vi "Host_Main.vi"() -> ()   [LabVIEW 2016]
uses:
  <extravilib>/ChannelInstances/Tag-bool/Write With Abort.vi
  <extravilib>/ChannelInstances/High Speed Stream-a[.](u8)/Instantiate.vi
  <extravilib>/ChannelInstances/Tag-bool/Instantiate.vi
  <extravilib>/ChannelInstances/Stream-wfm(dbl)/Instantiate.vi
  <extravilib>/ChannelInstances/Tag-bool/Endpoint.vi
  <vilib>/rtlsdr/rtlsdr.lvlib
  <extravilib>/ChannelInstances/Tag-bool.lvlib
panel:
  in  "stop":bool
  in  "Tuned Frequency (MHz)":u32=101000000 min=87000000 max=105000000 step=100000 format="%.1p"
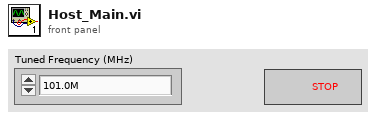
[diagram p1: front panel]
types:
  T1 = typedef "Tag-bool.lvlib/))Channel.ctl" = refnum<queue>
  T2 = typedef "High Speed Stream-a[.](u8).lvlib/)Channel.ctl" = refnum<queue>
  T3 = typedef "Stream-wfm(dbl).lvlib/)Channel.ctl" = refnum<queue>
  T4 = enum32{"invalid app kind", "Development System", "Run Time System", "Student Edition", "Embedded LabVIEW", "Evaluation", "Custom"}
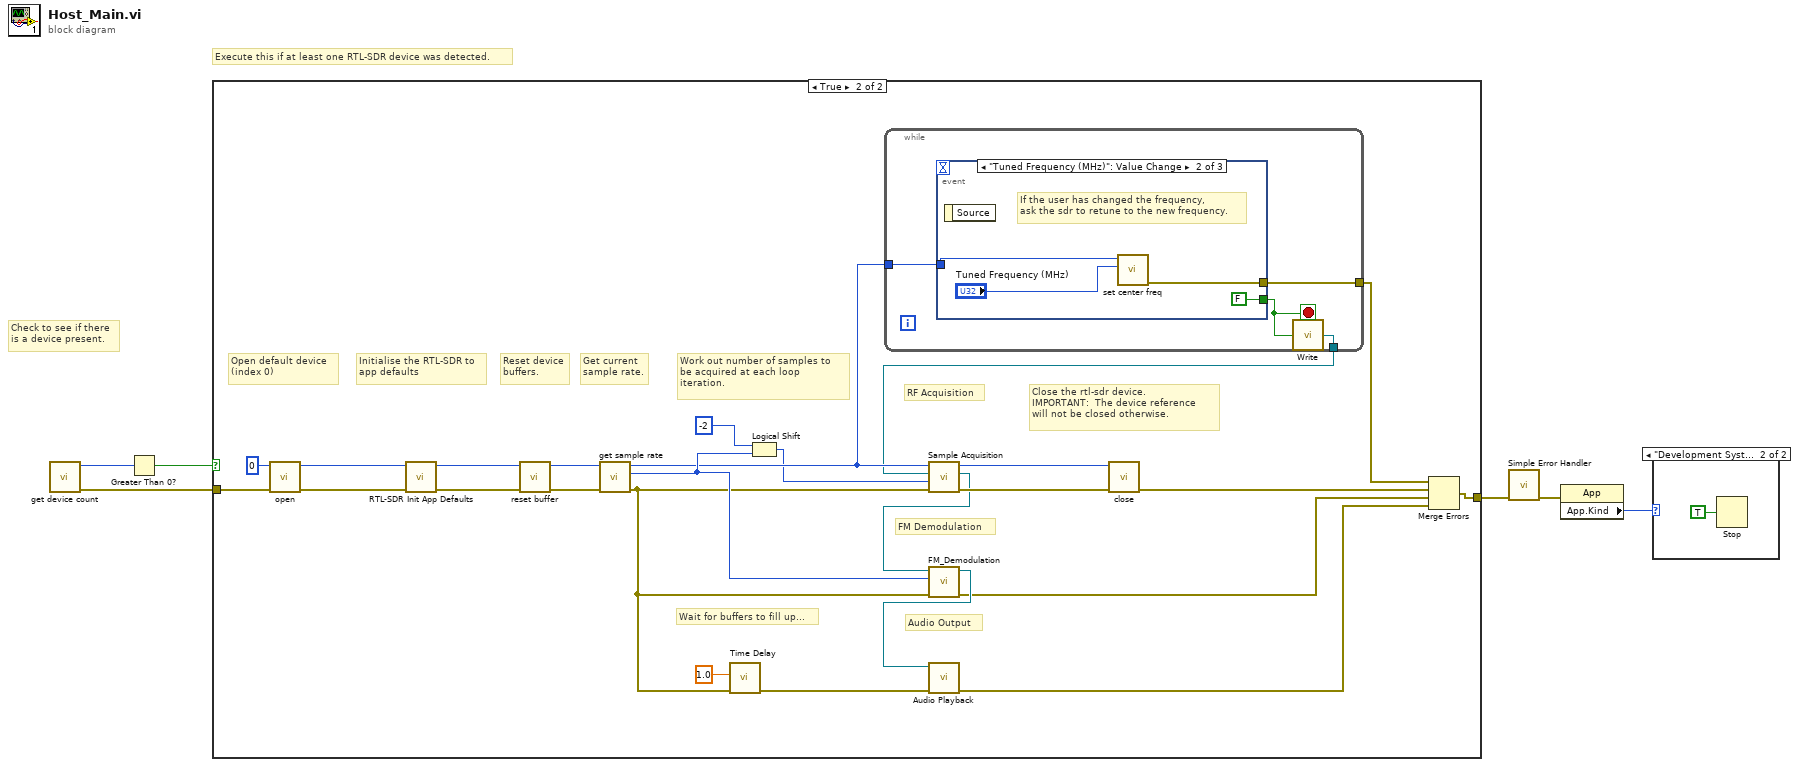
[diagram p0: block diagram]
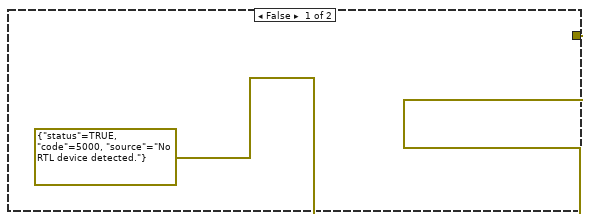
[diagram p2: hidden frame]
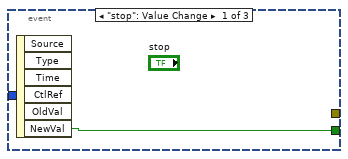
[diagram p3: hidden frame]
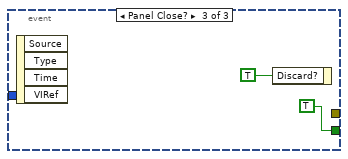
[diagram p4: hidden frame]
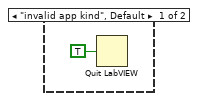
[diagram p5: hidden frame]
diagram:
  # "Execute this if at least one RTL-SDR device was detected."
  # "Check to see if there\nis a device present."
  n1 = call <vilib>:"get device count.vi"() -> ("error out"=w5:errorcluster, "Device Count"=w4:u32)  [unwired: 10 in]
  n2 = Greater Than 0?(x=w4) -> (x > 0?=w3:bool)
  n3 = case shown="True" w3 {
    tunnel: [errorcluster {"status"=TRUE, "code"=5000, "source"="No RTL device detected."} ("error out") w19] -> w6
    tunnel: w5 -> [_ w30]
    frame False {
    }
    frame True {
      # "Wait for buffers to fill up..."
      # "RF Acquisition"
      # "Audio Output"
      # "FM Demodulation"
      # "Reset device\nbuffers."
      # "Get current\nsample rate."
      # "Initialise the RTL-SDR to\napp defaults"
      # "Work out number of samples to\nbe acquired at each loop\niteration."
      # "Close the rtl-sdr device.\nIMPORTANT:  The device reference\nwill not be closed otherwise."
      # "Open default device\n(index 0)"
      n4 = call <vilib>:"open.vi"("error in (no error)"=w30, "Device Index"=u32 0 ("index")) -> ("error out"=w28:errorcluster, "DeviceRefnum Out"=w27:u64)  [unwired: 6 in]
      n5 = call "RTL-SDR Init App Defaults.vi"("error in (no error)"=w28, "RTL-SDR Device In"=w27) -> ("error out"=w26:errorcluster, "RTL-SDR Device Out"=w25:u64)  [unwired: 8 in]
      n6 = call <vilib>:"reset buffer.vi"("error in (no error)"=w26, "DeviceRefnum"=w25) -> ("error out"=w24:errorcluster, "DeviceRefnum Out"=w23:u64)  [unwired: 7 in, 1 out]
      n7 = call <vilib>:"get sample rate.vi"("error in (no error)"=w24, "DeviceRefnum"=w23) -> ("error out"=w10:errorcluster, "Sample Rate (Hz)"=w18:u32, "DeviceRefnum Out"=w16:u64)  [unwired: 7 in]
      n8 = call "Time Delay"("error in (no error)"=w10, "Delay Time (s)"=1.0) -> ("error out"=w9:errorcluster)  [unwired: 9 in]
      n9 = Logical Shift(y=i8 -2, x=w18) -> (x << y=w14:u32)
      n10 = while {
        tunnel: w16 -> [w36]
        tunnel: [w34] -> w15
        tunnel: [w33] -> w11
        stop <- w35 stop-if-true
        n11 = event shown="[1] \"Tuned Frequency (MHz)\": Value Change" {
          selector: _ -> [_ _ _]
          dyn-events: _ -> [_ _ _]
          timeout: _ -> [_ _ _]
          tunnel: w36 -> [_ w41 _]
          tunnel: [w37 FALSE ("NewVal") TRUE ("NewVal")] -> w35
          tunnel: [_ w38 _] -> w33
          event "stop": Value Change {
            n12 = event-data() -> ("NewVal"=w37:bool)  [unwired: 1 in, 5 out]
          }
          event "Tuned Frequency (MHz)": Value Change {
            # "If the user has changed the frequency,\nask the sdr to retune to the new frequency."
            n13 = event-data() -> ()  [unwired: 1 in, 1 out]
            n14 = call <vilib>:"set center freq.vi"("Center Frequency"="Tuned Frequency (MHz)", "DeviceRefnum"=w41) -> ("error out"=w38:errorcluster)  [unwired: 7 in, 2 out]
          }
          event Panel Close? {
            n15 = event-data() -> ()  [unwired: 1 in, 4 out]
            n16 = event-data("Discard?"=TRUE) -> ()  [unwired: 1 in, 1 out]
          }
        }
        n17 = call <extravilib>:"Write.vi"("element"=w35) -> ("channel"=w34:T1)  [unwired: 1 out]
      }
      n18 = call "Sample Acquisition.vi"("error in (no error)"=w10, "Samples per Read"=w14, "Channel in"=w15, "DeviceRefnum Out in"=w16) -> ("error out"=w31:errorcluster, "Channel out"=w13:T2, "DeviceRefnum Out out"=w12:u64)  [unwired: 5 in]
      n19 = call "FM_Demodulation.vi"("error in (no error)"=w10, "Sample Rate (Hz)"=w18, "Baseband Channel"=w13) -> ("error out"=w21:errorcluster, "Audio Channel Out"=w29:T3)  [unwired: 7 in]
      n20 = call "Audio Playback.vi"("error in (no error)"=w9, "Channel in"=w29) -> ("error out"=w22:errorcluster)  [unwired: 9 in]
      n21 = call <vilib>:"close.vi"("error in (no error)"=w31, "DeviceRefnum"=w12) -> ("error out"=w20:errorcluster)  [unwired: 8 in, 1 out]
      n22 = Merge Errors(w11, w20, w21, w22) -> (w19:errorcluster)
    }
  }
  n23 = call <vilib>:"Simple Error Handler.vi"("error in (no error)"=w6) -> ("error out"=w2:errorcluster)  [unwired: 4 in, 4 out]
  n24 = property class="App"(error in=w2) -> ("App.Kind"=w1:T4)  [unwired: 1 in, 2 out]
  n25 = case shown="\"Development System\"" w1 {
    frame "invalid app kind", Default {
      n26 = Quit LabVIEW(quit? (T)=TRUE) -> ()
    }
    frame "Development System" {
      n27 = Stop(stop? (T)=TRUE) -> ()
    }
  }
